vi "WriteSetting float.vi"(7 "value":dbl, 8 "error in (no error)":errorcluster, 10 "FPGA Setting":T1, 11 "FpgaRefBase in":refnum<class "FpgaRefBase.lvclass">) -> (0 "error out":errorcluster, 3 "FpgaRefBase out":refnum<class "FpgaRefBase.lvclass">)   [LabVIEW 2018, in "FpgaRefBase.lvclass"]
uses:
  FpgaRefBase.lvclass
  FPGA/fpga_settings.ctl
  <vilib>/Utility/error.llb/Error Cluster From Error Code.vi
  <vilib>/rvi/errors/niLvFpgaAdjustHostInterfaceError.vi
  <vilib>/rvi/FXPMathLib/FxpInterpret/XNode/nifxpmath_Interpret.xnode
  <vilib>/rvi/interface/nirviMethod/nirviMethod.xnode
  Scope/controls/settingsFPGAref.ctl
  <vilib>/FPGAPlugInAG/Dynamic/niLvFpga_WriteFifo_Dynamic.vi
  <vilib>/rvi/errors/niLvFpgaMergeErrorWithErrorCode.vi
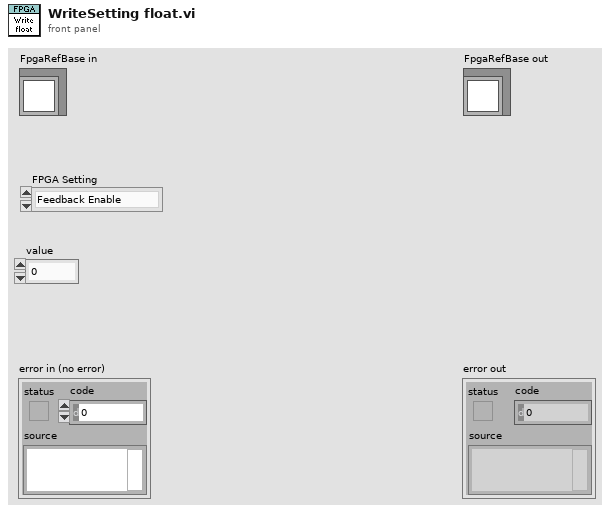
[diagram p1: front panel]
types:
  T1 = typedef "fpga_settings.ctl" = enum16{"Feedback Enable", "New FIR coeffs", "FIR shift", "Enable filter", "Set Downsample", "Downsample", "CIC Gain", "Record length", "Trigger samples", "Quiet time", "a_am", "b_am", "Use fixed delay", "fixed sin_fi", "fixed cos_fi", "Ki*Tau", "Kp", "Kd_Tau", "Fi_start", "Fi_delta", "DC_offs 0", "DC_offs 1", "DC_offs 2", "DC_offs 3", "Ki*Tau am", "Kp am", "Kd_Tau am", "Feedback AM", "Trigger delay", "Feedback delay", "Setpoint enable", "Beam enable", "Samples to acquire", "Cavity Enable", "Cavity C1", "Cavity C2", "Cavity C3", "Cavity C4", "Cavity C5"}
  T2 = typedef "settingsFPGAref.ctl" = refnum<k20>
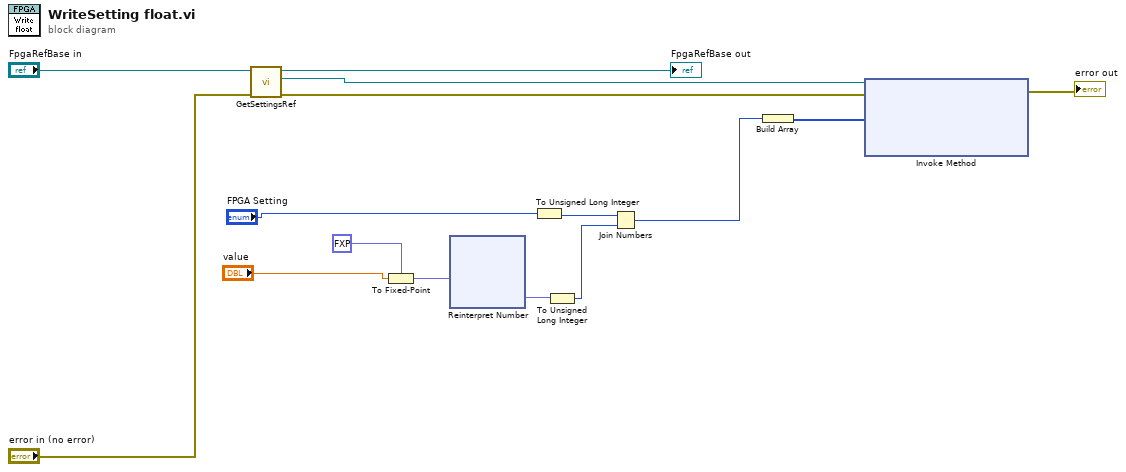
[diagram p0: block diagram]
diagram:
  n1 = call-dynamic "GetSettingsRef.vi"("error in (no error)"="error in (no error)", "FpgaRefBase in"="FpgaRefBase in") -> ("error out"=w2:errorcluster, "Settings FPGA ref"=w12:T2, "FpgaRefBase out"=→"FpgaRefBase out":refnum<class "FpgaRefBase.lvclass">)  [unwired: 7 in]
  n2 = To Fixed-Point(fixed-point type=fxp<+/-,32,4> 0.0 ("x"), number="value") -> (fixed-point=w10:fxp<+/-,32,4>)
  n3 = xnode "Reinterpret Number"("x"=w10) -> ("y"=w11:fxp<+,32,32>)
  n4 = To Unsigned Long Integer(number="FPGA Setting") -> (unsigned 32bit integer=w6:u32)
  n5 = To Unsigned Long Integer(number=w11) -> (unsigned 32bit integer=w5:u32)
  n6 = Join Numbers(hi=w6, lo=w5) -> ((hi.lo)=w4:u64)
  n7 = Build Array(w4) -> (w3:u64[])
  n8 = xnode "Invoke Method"("FPGA VI Reference In"=w12, "error in"=w2, "Data"=w3) -> ("error out"=→"error out":errorcluster)  [unwired: 1 in, 2 out]
